vi "Zmienna Globalna.vi"() -> ()   [LabVIEW 2020]
panel:
  in  "Tempo":dbl
  in  "Dane":dbl
  in  "stop":bool
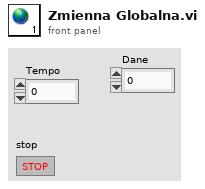
[diagram p1: front panel]
diagram:
